vi "Save Data.vi"(1 "error in (no error)":errorcluster, 2 "History Data":T1) -> (0 "error out":errorcluster)   [LabVIEW 2021]
doc: "Este VI guarda los datos pasados en el cluster de entrada en un fichero datalog"
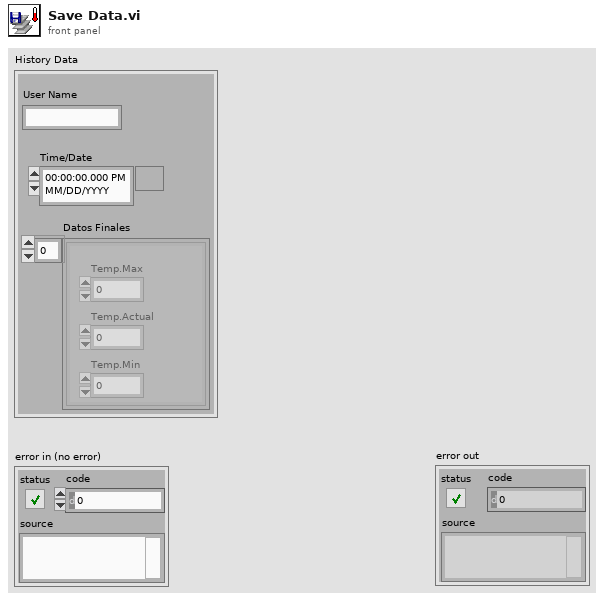
[diagram p1: front panel]
types:
  T1 = cluster{"User Name":string, "Time/Date":timestamp, "Datos Finales":cluster{"Temp.Max":dbl, "Temp.Actual":dbl, "Temp.Min":dbl}[]}
  T2 = enum16{"open", "replace", "create", "open or create", "replace or create", "replace or create with confirmation"}
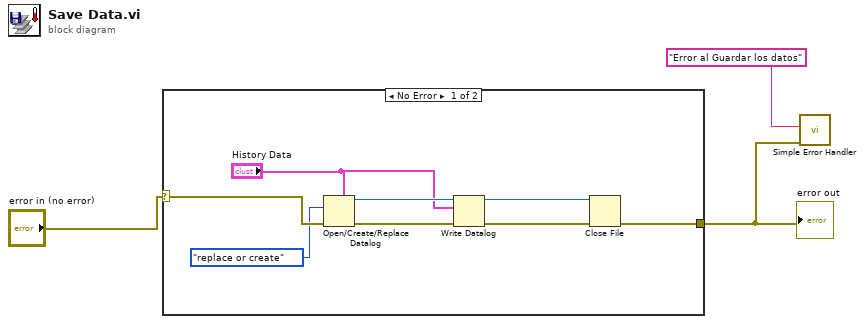
[diagram p0: block diagram]
diagram:
  n1 = case shown="No Error" "error in (no error)" {
    selector: "error in (no error)" -> [w8 w12]
    tunnel: [w5 w12] -> w3
    frame No Error {
      n2 = Open/Create/Replace Datalog(5:"History Data", 8:w8, 10:T2."replace or create" ("operation (0:open)")) -> (0:w7:errorcluster, 3:w11:refnum<k1>)  [unwired: 3 in, 1 out]
      n3 = Write Datalog(4:w7, 6:"History Data", 7:w11) -> (0:w6:errorcluster, 3:w10:refnum<k1>)
      n4 = Close File(refnum=w10, error in=w6) -> (error out=w5:errorcluster)  [unwired: 1 out]
    }
    frame Error {
    }
  }
  "error out" <- w3
  n5 = call <vilib>:"Simple Error Handler.vi"("error source (\" \")"="Error al Guardar los datos" ("error source (\" \")"), "error in (no error)"=w3) -> ()  [unwired: 3 in, 5 out]
